vi "Register LabVIEW Application.vi"   [LabVIEW 2015, in "Reaper.lvclass"]
uses:
  Reaper.lvclass
  Reaper.lvclass/Reaper.ctl
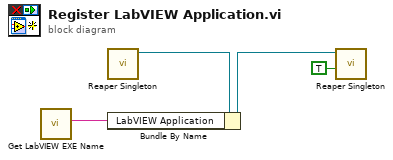
[diagram p0: block diagram]
diagram:
  n1 = call "Get LabVIEW EXE Name.vi"() -> ("LabVIEW EXE Name"=w1:string)  [unwired: 11 in]
  n2 = call "Reaper Singleton.vi"() -> ("Reaper Out"=w3:refnum<class "Reaper.lvclass">)  [unwired: 11 in]
  n3 = Bundle By Name(cluster=w3, "LabVIEW Application"=w1) -> (w4:refnum<class "Reaper.lvclass">)
  n4 = call "Reaper Singleton.vi"("Write? (F)"=TRUE, "Reaper In"=w4) -> ()  [unwired: 9 in, 1 out]
